vi "main vi.vi"() -> ()   [LabVIEW 2020]
uses:
  System.Speech
panel:
  in  "Read":bool
  out "text":string
  in  "file path (use dialog)":path
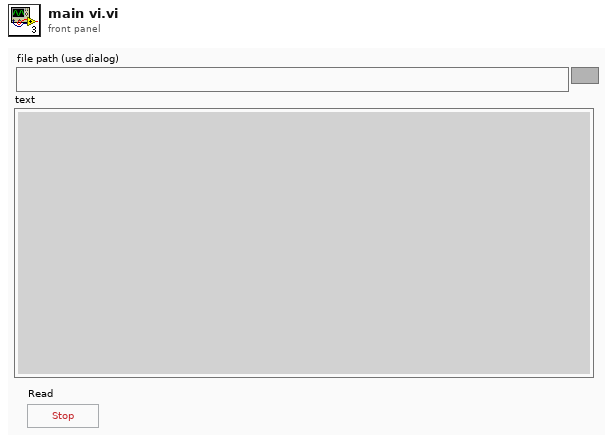
[diagram p1: front panel]
types:
  T1 = enum16{"open", "replace", "create", "open or create", "replace or create", "replace or create with confirmation"}
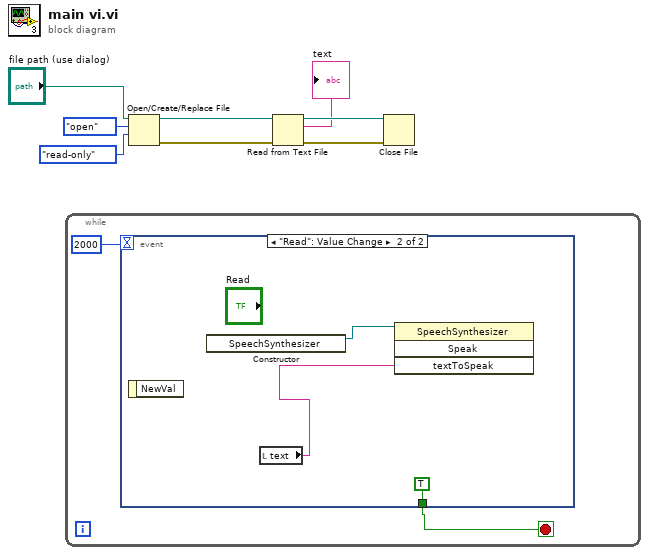
[diagram p0: block diagram]
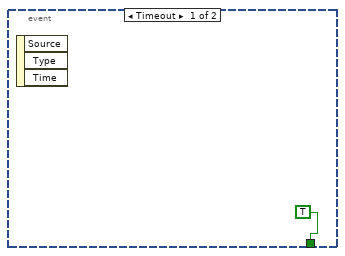
[diagram p2: hidden frame]
diagram:
  n1 = while {
    stop <- w9 stop-if-true
    n2 = event shown="[1] \"Read\": Value Change" {
      selector: _ -> [_ _]
      dyn-events: _ -> [_ _]
      timeout: 2000 -> [_ _]
      tunnel: [TRUE TRUE] -> w9
      event Timeout {
        n3 = event-data() -> ()  [unwired: 1 in, 3 out]
      }
      event "Read": Value Change {
        n4 = event-data() -> ()  [unwired: 1 in, 1 out]
        n5 = constructor class="SpeechSynthesizer"() -> (reference out=w13:refnum<k24>)  [unwired: 3 in, 2 out]
        n6 = local read "text"() -> (w14:string)
        n7 = invoke class="SpeechSynthesizer" method="Speak"(reference=w13, "textToSpeak"=w14) -> ()  [unwired: 2 in, 4 out]
      }
    }
  }
  n8 = Open/Create/Replace File(file path (use dialog)="file path (use dialog)", operation (0:open)=T1."open", access (0:read/write)=enum16{"read/write", "read-only", "write-only"}."read-only") -> (refnum out=w8:refnum<file>, error out=w6:errorcluster)  [unwired: 3 in, 1 out]
  n9 = Read from Text File(file (use dialog)=w8, error in=w6) -> (refnum out=w7:refnum<file>, text=→"text":string, error out=w5:errorcluster)  [unwired: 2 in, 1 out]
  n10 = Close File(refnum=w7, error in=w5) -> ()  [unwired: 2 out]
